vi "CSV To Dictionary.vi"(0 "CSV String":string, 5 "Header? (False)":bool, 11 "Error in":errorcluster caption="Error in (no error)") -> (4 "Dictionary":refnum<class "Dictionary.lvclass">, 15 "Error out":errorcluster)   [LabVIEW 2018, in "Dictionary - CSV.lvlib"]
doc: "Creates a new <B>Dictionary</B> with the contents of <B>CSV String</B> loaded into it.\n\nMapping of <B>CSV String</B> to <B>Dictionary</B>:\n- CSV fields names will become top level dictionaries.\n- CSV values are stored as strings. Enclosing quotes will be removed.\n- Dictionary entities are added to field names.\n\nThis VI runs only if there is no error on <B>Error in</B>.\n\nKåre Juul Kirkegaard\nGPower\n4/4 2019"
uses:
  Dictionary - CSV.lvlib
  <vilib>/GPower/Dictionary/Library/Dictionary Class/Dictionary.lvclass
  <vilib>/Utility/error.llb/whitespace.ctl
  bff844dc-819a-48d8-9d4a-e148e280f49e.vi
  <vilib>/GPower/Dictionary/Library/Dictionary Class/Set/Set Or Append Value.vi
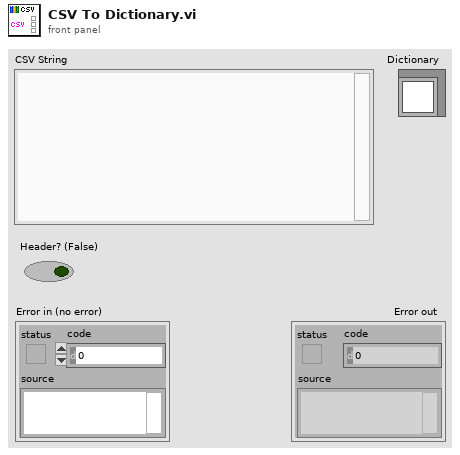
[diagram p1: front panel]
types:
  T1 = typedef "whitespace.ctl" = u16
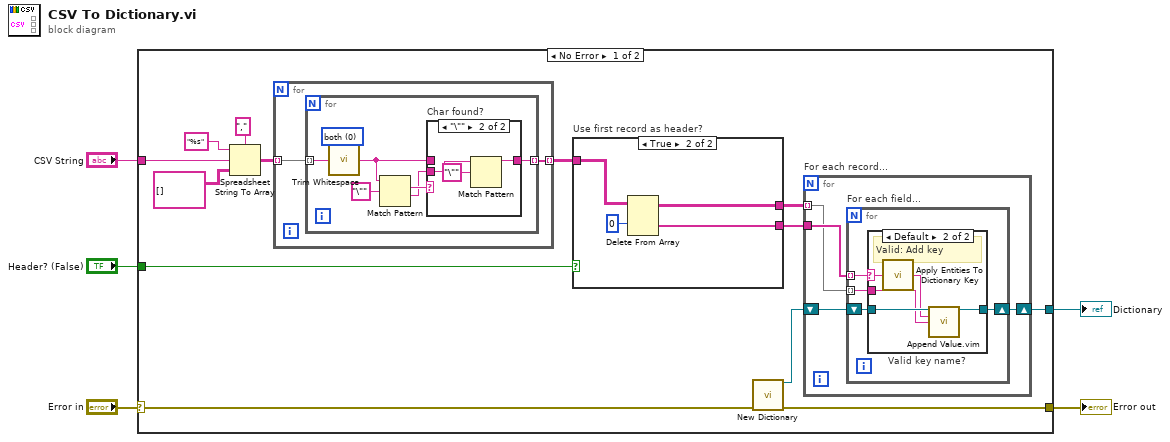
[diagram p0: block diagram]
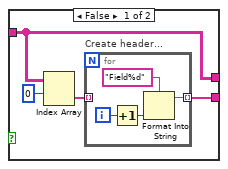
[diagram p3: hidden frame]
diagram:
  n1 = case shown="No Error" "Error in" {
    selector: "Error in" -> [w18 w58]
    tunnel: [w17 w58] -> w1
    tunnel: "CSV String" -> [w9 _]
    tunnel: "Header? (False)" -> [w8 _]
    tunnel: [w15 _] -> w2
    frame No Error {
      n2 = Spreadsheet String To Array(delimiter (Tab)=",", format string="%s", spreadsheet string=w9, array type (2D Dbl)=string[][] []) -> (array=w10:string[][])
      n3 = for {
        tunnel: w10 -> [w46] mode=indexing
        tunnel: [w45] -> w7 mode=indexing
        n4 = for {
          tunnel: w46 -> [w53] mode=indexing
          tunnel: [w48] -> w45 mode=indexing
          w52 = T1 0 items=["both", "start of string", "end of string"] ("location (both)")
          n5 = call <vilib>:"Trim Whitespace.vi"("string"=w53, "location (both)"=w52) -> ("trimmed string"=w49:string)
          n6 = Match Pattern(string=w49, regular expression="\"") -> (match substring=w50:string, after substring=w47:string)  [unwired: 1 in, 2 out]
          n7 = case "Char found?" shown="\"\\\"\"" w50 {
            tunnel: w49 -> [w54 _]
            tunnel: w47 -> [_ w56]
            tunnel: [w54 w55] -> w48
            frame Default {
            }
            frame "\"" {
              n8 = Match Pattern(string=w56, regular expression="\"") -> (before substring=w55:string)  [unwired: 1 in, 3 out]
            }
          }
        }
      }
      n9 = case "Use first record as header?" shown="True" w8 {
        tunnel: [w36 w41] -> w14
        tunnel: w7 -> [w33 w44]
        tunnel: [w33 w42] -> w6
        frame False {
          n10 = Index Array(array=w33, index (row)=0) -> (element=w34:string[])  [unwired: 1 in]
          n11 = for "Create header..." {
            tunnel: [w37] -> w36 mode=indexing
            tunnel: w34 -> [_] mode=indexing
            i -> [w39]
            n12 = Increment(x=w39) -> (x+1=w38:i32)
            n13 = Format Into String(format string="Field%d", w38) -> (resulting string=w37:string)  [unwired: 2 in, 1 out]
          }
        }
        frame True {
          n14 = Delete From Array(array=w44, index (row)=0) -> (deleted portion=w41:string[], array with subset deleted=w42:string[][])  [unwired: 2 in]
        }
      }
      n15 = call <vilib>:"New Dictionary.vi"("Error in"=w18) -> ("New Dictionary"=w16:refnum<class "Dictionary.lvclass">, "Error out"=w17:errorcluster)  [unwired: 13 in]
      n16 = for "For each record..." {
        tunnel: w14 -> [w20]
        shift-right: [w21] -> w15
        shift-left: w16 -> [w22]
        tunnel: w6 -> [w19] mode=indexing
        n17 = for "For each field..." {
          shift-right: [w25] -> w21
          shift-left: w22 -> [w26]
          tunnel: w20 -> [w23] mode=indexing
          tunnel: w19 -> [w24] mode=indexing
          n18 = case "Valid key name?" shown="Default" w23 {
            selector: w23 -> [_ w28]
            tunnel: w26 -> [w27 w32]
            tunnel: w24 -> [_ w31]
            tunnel: [w27 w30] -> w25
            frame "" {
              # "Invalid: Skip key"
            }
            frame Default {
              # "Valid: Add key"
              n19 = call <vilib>:"Apply Entities To Dictionary Key.vi"("Clear Dictionary Key"=w28) -> ("Encoded Dictionary Key"=w29:string)
              n20 = call "Append Value.vim"("Dictionary in"=w32, "Requested Key Path"=w29, "Value"=w31) -> ("Dictionary out"=w30:refnum<class "Dictionary.lvclass">)  [unwired: 10 in, 2 out]
            }
          }
        }
      }
    }
    frame Error {
    }
  }
  "Error out" <- w1
  "Dictionary" <- w2
